vi "18_TCP_READ_WRITE_COVID_19.vi"() -> ()   [LabVIEW 2019]
panel:
  out "bytes written":i32
  in  "data in":string
  out "connection ID 2":refnum<k5>
  in  "WRITE":bool
  out "net address":u32
  in  "stop":bool
  out "data out":string
  out "connection ID":refnum<k5>
  in  "mode (standard)":T1(ring)
  in  "bytes to read":i32
  out "remote port":u16
  out "remote address":string
  # "ESCRITURA"
  # "LECTURA"
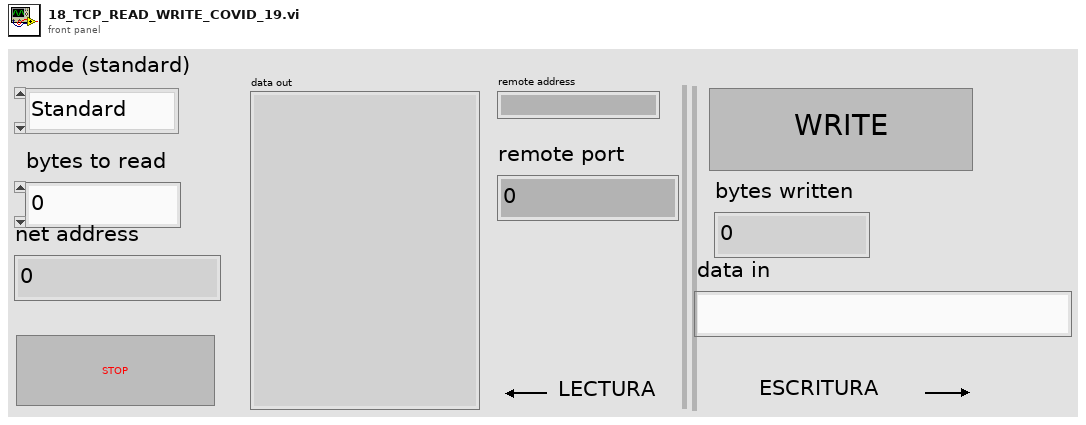
[diagram p1: front panel]
types:
  T1 = enum16{"Standard", "Buffered", "CRLF", "Immediate"}
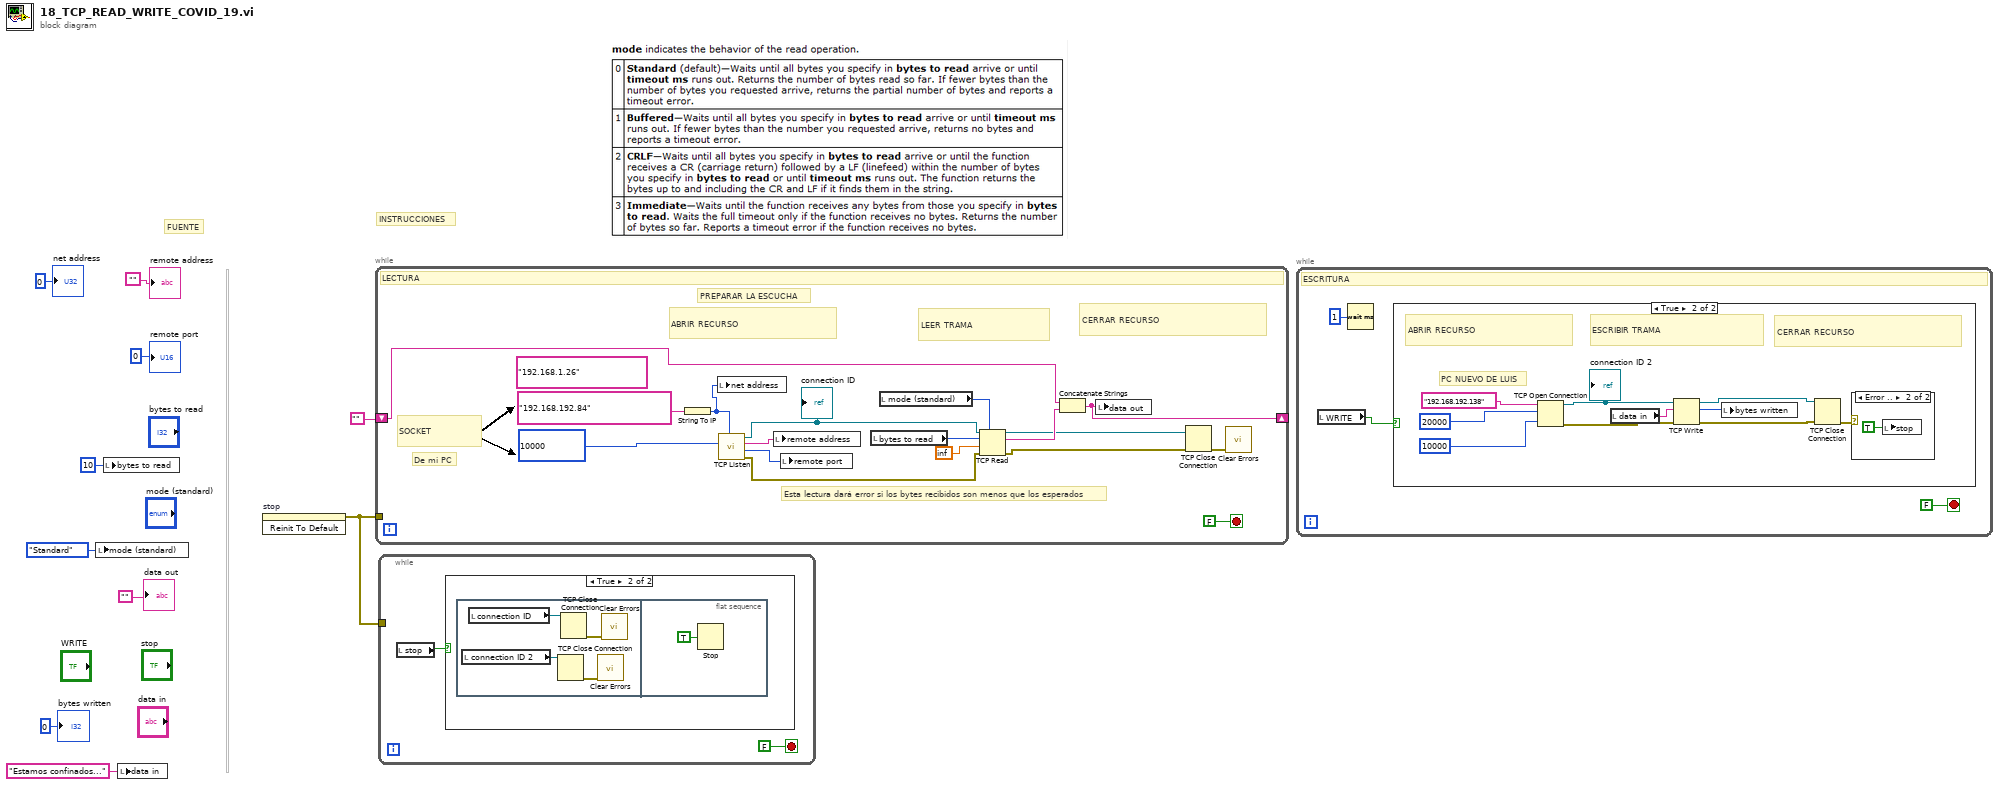
[diagram p0: block diagram]
diagram:
  # "INSTRUCCIONES"
  # "FUENTE"
  n1 = local write "mode (standard)"(T1."Standard" ("mode (standard)")) -> ()
  n2 = local write "bytes to read"(10 ("bytes to read")) -> ()
  n3 = local write "data in"("Estamos confinados..." ("data in")) -> ()
  n4 = invoke on="stop" class="Bool (strict)" method="Reinit To Default"() -> (error out=w5:errorcluster)  [unwired: 3 in, 2 out]
  n5 = while {
    shift-right: [w17] -> _
    shift-left: "" -> [w16]
    tunnel: w5 -> [_]
    stop <- FALSE stop-if-true
    (unwired) "192.168.1.26" ("name")
    # "De mi PC"
    # "CERRAR RECURSO"
    # "Esta lectura dará error si los bytes recibidos son menos que los esperados"
    # "LEER TRAMA"
    # "SOCKET"
    # "ABRIR RECURSO"
    # "PREPARAR LA ESCUCHA"
    # "LECTURA"
    n6 = String To IP(1:"192.168.192.84" ("name")) -> (0:w11:u32)
    n7 = local write "net address"(w11) -> ()
    n8 = call <vilib>:"TCP Listen.vi"("net address"=w11, "port"=u16 10000) -> ("error out"=w22:errorcluster, "remote port"=w24:u16, "remote address"=w25:string, "connection ID"=w23:refnum<k5>)  [unwired: 5 in, 1 out]
    "connection ID" <- w23
    n9 = local write "remote address"(w25) -> ()
    n10 = local write "remote port"(w24) -> ()
    n11 = local read "bytes to read"() -> (w20:i32)
    n12 = local read "mode (standard)"() -> (w19:T1)
    n13 = TCP Read(connection ID=w23, bytes to read=w20, error in (no error)=w22, 7:w19, 9:inf) -> (connection ID out=w14:refnum<k5>, data out=w15:string, error out=w13:errorcluster)
    n14 = Concatenate Strings(w16, w15) -> (w17:string)
    n15 = local write "data out"(w17) -> ()
    n16 = TCP Close Connection(connection ID=w14, error in (no error)=w13) -> (error out=w12:errorcluster)  [unwired: 1 in, 1 out]
    n17 = call <vilib>:"Clear Errors.vi"("error in (no error)"=w12) -> ()  [unwired: 5 in, 2 out]
  }
  n18 = while {
    tunnel: w5 -> [_]
    stop <- FALSE stop-if-true
    n19 = local read "stop"() -> (w28:bool)
    n20 = case shown="True" w28 {
      frame False {
      }
      frame True {
        n21 = flat-sequence {
          frame #0 {
            n22 = local read "connection ID 2"() -> (w31:refnum<k5>)
            n23 = local read "connection ID"() -> (w32:refnum<k5>)
            n24 = TCP Close Connection(connection ID=w31) -> (error out=w30:errorcluster)  [unwired: 2 in, 1 out]
            n25 = TCP Close Connection(connection ID=w32) -> (error out=w33:errorcluster)  [unwired: 2 in, 1 out]
            n26 = call <vilib>:"Clear Errors.vi"("error in (no error)"=w30) -> ()  [unwired: 5 in, 2 out]
            n27 = call <vilib>:"Clear Errors.vi"("error in (no error)"=w33) -> ()  [unwired: 5 in, 2 out]
          }
          frame #1 {
            n28 = Stop(stop? (T)=TRUE) -> ()
          }
        }
      }
    }
  }
  n29 = while {
    stop <- FALSE stop-if-true
    # "ESCRITURA"
    n30 = local read "WRITE"() -> (w36:bool)
    n31 = Wait (ms)(milliseconds to wait=u32 1) -> ()  [unwired: 1 out]
    n32 = case shown="True" w36 {
      frame False {
      }
      frame True {
        # "PC NUEVO DE LUIS"
        # "CERRAR RECURSO"
        # "ESCRIBIR TRAMA"
        # "ABRIR RECURSO"
        n33 = TCP Open Connection(address="192.168.192.138", remote port or service name=u16 20000, local port=u16 10000 ("local port (0)")) -> (connection ID=w44:refnum<k5>, error out=w43:errorcluster)  [unwired: 2 in]
        "connection ID 2" <- w44
        n34 = local read "data in"() -> (w42:string)
        n35 = TCP Write(connection ID=w44, data in=w42, error in (no error)=w43) -> (connection ID out=w40:refnum<k5>, bytes written=w41:i32, error out=w39:errorcluster)  [unwired: 1 in]
        n36 = local write "bytes written"(w41) -> ()
        n37 = TCP Close Connection(connection ID=w40, error in (no error)=w39) -> (error out=w38:errorcluster)  [unwired: 1 in, 1 out]
        n38 = case shown="Error .." w38 {
          frame No Error {
          }
          frame Error {
            n39 = local write "stop"(TRUE ("stop")) -> ()
          }
        }
      }
    }
  }
  "remote address" <- ""
  "remote port" <- u16 0
  "data out" <- ""
  "net address" <- u32 0 ("net address")
  "bytes written" <- 0 ("bytes written")
